vi "Keithley 6221 DC Block Continuous with Stim Trigger.vi"() -> ()   [LabVIEW 2020]
uses:
  <instrlib>/Keithley 622x LV 2009/Utility/Typedefs/KE622x -- Instrument Type.ctl
  <instrlib>/Keithley 622x LV 2009/Typedefs/KE622x -- On Off Control.ctl
  <instrlib>/Keithley 622x LV 2009/Configure/Output/Typedefs/KE6221 -- Output Response.ctl
  <instrlib>/Keithley 622x LV 2009/Configure/Source/Typedefs/KE622x -- Current Range.ctl
  <instrlib>/Keithley 622x LV 2009/Configure/Source/Typedefs/KE622x -- Current Ranges.ctl
  <instrlib>/Keithley 622x LV 2009/Configure/Source/Typedefs/KE622x -- Voltage Limit.ctl
  <instrlib>/Keithley 622x LV 2009/Utility/Typedefs/KE622x -- Serial Port Settings.ctl
  <instrlib>/Keithley 622x LV 2009/Configure/Source/Typedefs/KE622x -- Current Level.ctl
  <vilib>/DAQmx/write.llb/DAQmx Write (Analog 1D DBL 1Chan NSamp).vi
  <vilib>/DAQmx/create/channels.llb/DAQmx Create Channel (AO-Voltage-Basic).vi
  <vilib>/DAQmx/configure/timing.llb/DAQmx Timing (Sample Clock).vi
  <vilib>/DAQmx/miscellaneous.llb/DAQmx Fill In Error Info.vi
  <instrlib>/Keithley 622x LV 2009/Keithley 622x.lvlib
panel:
  in  "Keithley COM Port":refnum<visa-resource-name>
  in  "Block\nAmplitude (mA)":dbl=1.0
  in  "stop":bool
  in  "NI DAQ Trigger Channel":tag
  in  "Pulse\nFrequency (Hz)":dbl=1.0 min=0.01 max=50.0
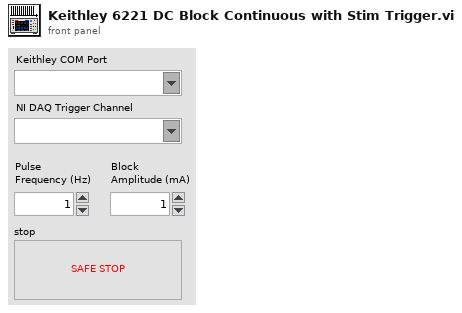
[diagram p1: front panel]
types:
  T1 = typedef "Keithley 622x.lvlib/KE622x -- On Off Control.ctl" = enum16{"Off", "On"}
  T2 = typedef "Keithley 622x.lvlib/KE622x -- Current Level.ctl" = dbl
  T3 = typedef "Keithley 622x.lvlib/KE622x -- Serial Port Settings.ctl" = cluster{"Read Term Char":enum16{"CR", "LF", "CR + LF", "LF + CR"}, "Baud Rate":enum16{"300", "600", "1200", "2400", "4800", "9600", "19200", "38400", "57600", "115200"}, "Flow Control\n(XON / XOFF)":enum16{"Off", "On"}}
  T4 = typedef "Keithley 622x.lvlib/KE622x -- Voltage Limit.ctl" = dbl
  T5 = typedef "Keithley 622x.lvlib/KE622x -- Current Range.ctl" = cluster{"Auto Range?":bool, "Man / Selected\nRange":T6}
  T6 = typedef "Keithley 622x.lvlib/KE622x -- Current Ranges.ctl" = enum16{"2nA", "20nA", "200nA", "2uA", "20uA", "200uA", "2mA", "20mA", "100mA"}
  T7 = typedef "Keithley 622x.lvlib/KE6221 -- Output Response.ctl" = enum16{"Fast", "Slow"}
  T8 = typedef "Keithley 622x.lvlib/KE622x -- Instrument Type.ctl" = enum16{"KE6220", "KE6221"}
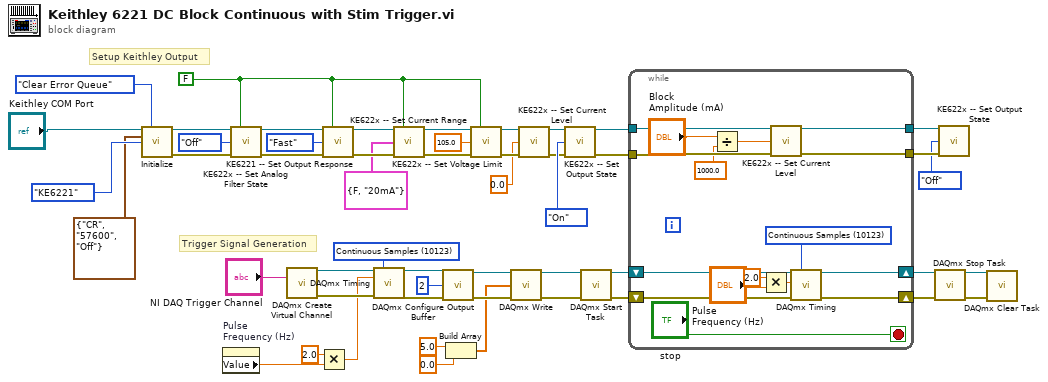
[diagram p0: block diagram]
diagram:
  w23 = FALSE ("Check For SCPI Errors? (T)")
  w46 = 10123 items=["Finite Samples"=10178, "Continuous Samples"=10123, "Hardware Timed Single Point"=12522] ("sample mode")
  # "Setup Keithley Output"
  # "Trigger Signal Generation"
  n1 = call <instrlib>:"Initialize.vi"("VISA resource name"="Keithley COM Port", "Error Queue Option"=enum16{"Clear Error Queue", "Error Query"}."Clear Error Queue", "RS-232 Settings"=T3 {"Read Term Char"=enum."CR", "Baud Rate"=enum."57600", "Flow Control\n(XON / XOFF)"=enum."Off"}, "Instrument Type"=KE622x_--_Instrument_Type."KE6221") -> ("VISA resource name out"=w33:refnum<visa-resource-name>, "error out"=w32:errorcluster)  [unwired: 10 in]
  n2 = property on="Pulse\nFrequency (Hz)" class="DigNum (strict)"() -> ("Value"=w2:dbl)  [unwired: 2 in, 2 out]
  n3 = call <instrlib>:"KE622x -- Set Analog Filter State.vi"("Resource In"=w33, "Check For SCPI Errors? (T)"=w23, "Analog Filter State"=KE622x_--_On_Off_Control."Off", "error in (no error)"=w32) -> ("Resource Out (dupl)"=w31:refnum<visa-resource-name>, "error out"=w30:errorcluster)  [unwired: 10 in]
  n4 = call-poly <vilib>:"DAQmx Create Virtual Channel.vi"("physical channels"="NI DAQ Trigger Channel") -> ("task out"=w48:refnum<k21>, "error out"=w47:errorcluster)  [unwired: 13 in]
  n5 = Multiply(x=2.0, y=w2) -> (x*y=w3:dbl)
  n6 = call <instrlib>:"KE6221 -- Set Output Response.vi"("Resource In"=w31, "Check For SCPI Errors? (T)"=w23, "KE6221 Output Response"=KE6221_--_Output_Response."Fast", "error in (no error)"=w30) -> ("Resource Out (dupl)"=w26:refnum<visa-resource-name>, "error out"=w25:errorcluster)  [unwired: 10 in]
  n7 = call-poly <vilib>:"DAQmx Timing.vi"("task/channels in"=w48, "sample mode"=w46, "rate"=w3, "error in"=w47) -> ("task out"=w44:refnum<k21>, "error out"=w43:errorcluster)  [unwired: 10 in]
  n8 = call <instrlib>:"KE622x -- Set Current Range.vi"("Resource In"=w26, "Check For SCPI Errors? (T)"=w23, "Current Range In"=T5 {"Auto Range?"=FALSE, "Man / Selected\nRange"=enum."20mA"}, "error in (no error)"=w25) -> ("Resource Out (dupl)"=w22:refnum<visa-resource-name>, "error out"=w21:errorcluster)  [unwired: 9 in, 1 out]
  n9 = call <vilib>:"DAQmx Configure Output Buffer.vi"("task/channels in"=w44, "buffer size (in samples per channel)"=u32 2, "error in"=w43) -> ("task out"=w42:refnum<k21>, "error out"=w41:errorcluster)  [unwired: 11 in]
  n10 = Build Array(5.0 ("element"), 0.0 ("element")) -> (w4:dbl[])
  n11 = call <instrlib>:"KE622x -- Set Voltage Limit.vi"("Resource In"=w22, "Check For SCPI Errors? (T)"=w23, "Voltage Limit (V)"=T4 105.0, "error in (no error)"=w21) -> ("Resource Out (dupl)"=w16:refnum<visa-resource-name>, "error out"=w15:errorcluster)  [unwired: 10 in]
  n12 = call-poly <vilib>:"DAQmx Write.vi"("task/channels in"=w42, "data"=w4, "error in"=w41) -> ("task out"=w40:refnum<k21>, "error out"=w35:errorcluster)  [unwired: 10 in, 1 out]
  n13 = call <instrlib>:"KE622x -- Set Current Level.vi"("Resource In"=w16, "Current Level (A) In"=T2 0.0, "error in (no error)"=w15) -> ("Resource Out (dupl)"=w17:refnum<visa-resource-name>, "error out"=w14:errorcluster)  [unwired: 10 in, 1 out]
  n14 = call <instrlib>:"KE622x -- Set Output State.vi"("Resource In"=w17, "Output State"=KE622x_--_On_Off_Control."On", "error in (no error)"=w14) -> ("Resource Out (dupl)"=w12:refnum<visa-resource-name>, "error out"=w11:errorcluster)  [unwired: 11 in]
  n15 = call <vilib>:"DAQmx Start Task.vi"("task/channels in"=w40, "error in"=w35) -> ("task out"=w38:refnum<k21>, "error out"=w37:errorcluster)  [unwired: 12 in]
  n16 = while {
    shift-right: [w58] -> w39
    shift-left: w38 -> [w53]
    shift-right: [w52] -> w36
    shift-left: w37 -> [w54]
    tunnel: w12 -> [w66]
    tunnel: w11 -> [w65]
    tunnel: [w64] -> w10
    tunnel: [w63] -> w9
    stop <- "stop" stop-if-true
    w59 = 10123 items=["Finite Samples"=10178, "Continuous Samples"=10123, "Hardware Timed Single Point"=12522] ("sample mode")
    n17 = Divide(x="Block\nAmplitude (mA)", y=1000.0) -> (x/y=w62:dbl)
    n18 = Multiply(x=2.0, y="Pulse\nFrequency (Hz)") -> (x*y=w56:dbl)
    n19 = call <instrlib>:"KE622x -- Set Current Level.vi"("Resource In"=w66, "Current Level (A) In"=w62, "error in (no error)"=w65) -> ("Resource Out (dupl)"=w64:refnum<visa-resource-name>, "error out"=w63:errorcluster)  [unwired: 10 in, 1 out]
    n20 = call-poly <vilib>:"DAQmx Timing.vi"("task/channels in"=w53, "sample mode"=w59, "rate"=w56, "error in"=w54) -> ("task out"=w58:refnum<k21>, "error out"=w52:errorcluster)  [unwired: 10 in]
  }
  n21 = call <vilib>:"DAQmx Stop Task.vi"("task/channels in"=w39, "error in"=w36) -> ("task out"=w51:refnum<k21>, "error out"=w50:errorcluster)  [unwired: 12 in]
  n22 = call <instrlib>:"KE622x -- Set Output State.vi"("Resource In"=w10, "Output State"=KE622x_--_On_Off_Control."Off", "error in (no error)"=w9) -> ()  [unwired: 11 in, 2 out]
  n23 = call <vilib>:"DAQmx Clear Task.vi"("task in"=w51, "error in"=w50) -> ()  [unwired: 13 in, 1 out]
